vi "UpdateVariable.vi"(8 "error in":errorcluster, 9 "compressed":bool, 10 "value in":string, 11 "variable":string) -> (0 "error out":errorcluster)   [LabVIEW 2011]
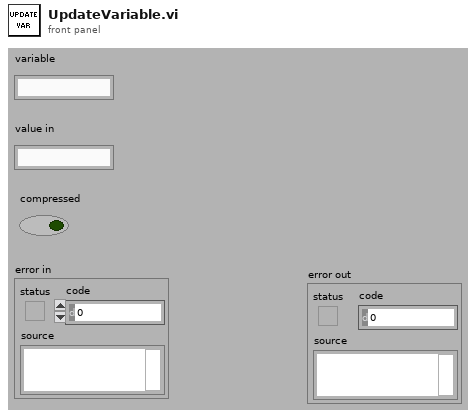
[diagram p1: front panel]
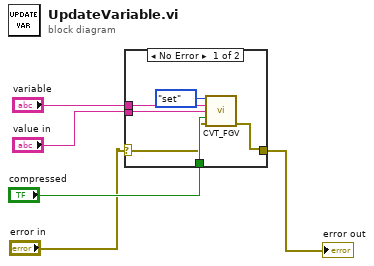
[diagram p0: block diagram]
diagram:
  n1 = case shown="No Error" "error in" {
    selector: "error in" -> [w7 w12]
    tunnel: "compressed" -> [w11 _]
    tunnel: "value in" -> [w10 _]
    tunnel: "variable" -> [w9 _]
    tunnel: [w6 w12] -> w1
    frame No Error {
      n2 = call "CVT_FGV.vi"("command"=enum16{"set", "get", "reset"}."set", "variable"=w9, "value in"=w10, "compressed"=w11, "error in"=w7) -> ("error out"=w6:errorcluster)  [unwired: 8 in, 2 out]
    }
    frame Error {
    }
  }
  "error out" <- w1
